vi "Handle Error.vi"(8 "error in (no error)":errorcluster, 11 "UI Wizard in":refnum<class "UI Wizard.lvclass">) -> (0 "error out":errorcluster, 2 "stop actor?":bool=TRUE, 3 "UI Wizard out":refnum<class "UI Wizard.lvclass">)   [LabVIEW 2013, in "SET Project Editor.lvlib" / "UI Wizard.lvclass"]
doc: "(<B>Filename</B>: Actor Framework.lvlib:Actor.lvclass:Handle Error.vi)\n\nDefines how the actor handles an error that occurred while processing a message.\n\nBy default, this method does nothing except stop the actor. This method also treats error code 43 (coming from <B>error in</B>) as a sign that the actor shut down normally. In this situation, the Handle Error method does not return the error on <B>error out</B>, meaning the actor's caller will not receive it. All other error codes will be returned on <B>error out</B>.\n\nA descendant class may override this method to change this behavior."
uses:
  UI Wizard.lvclass
  UI Actor/UI Actor.lvclass
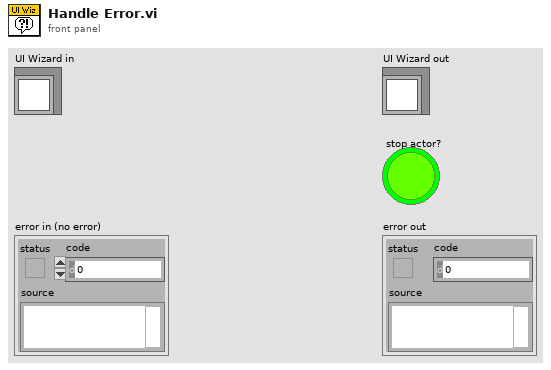
[diagram p1: front panel]
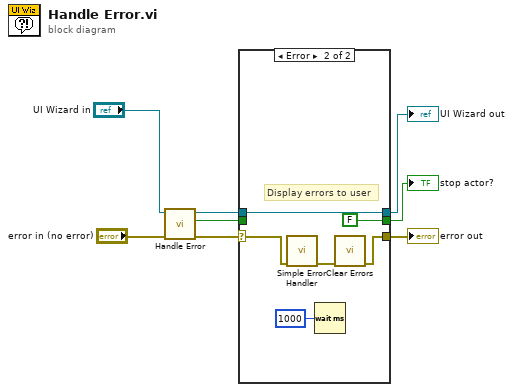
[diagram p0: block diagram]
diagram:
  n1 = call-parent "Handle Error.vi"("error in (no error)"="error in (no error)", "Actor in"="UI Wizard in") -> ("error out"=w5:errorcluster, "stop actor?"=w4:bool, "Actor out"=w6:refnum<class "UI Wizard.lvclass">)  [unwired: 7 in]
  n2 = case shown="Error" w5 {
    selector: w5 -> [w9 w15]
    tunnel: w4 -> [w10 _]
    tunnel: w6 -> [w11 w17]
    tunnel: [w11 w17] -> w3
    tunnel: [w10 FALSE ("stop actor?")] -> w2
    tunnel: [w9 w12] -> w1
    frame No Error {
    }
    frame Error {
      # "Display errors to user"
      n3 = call <vilib>:"Simple Error Handler.vi"("error in (no error)"=w15) -> ("error out"=w13:errorcluster)  [unwired: 4 in, 4 out]
      n4 = Wait (ms)(milliseconds to wait=u32 1000) -> ()  [unwired: 1 out]
      n5 = call <vilib>:"Clear Errors.vi"("error in (no error)"=w13) -> ("error out"=w12:errorcluster)  [unwired: 6 in]
    }
  }
  "UI Wizard out" <- w3
  "error out" <- w1
  "stop actor?" <- w2
